vi "MinerHash.vi"(3 "TimeDelay":u32=100, 4 "difficulty":i32=70001, 5 "expected":string="3BE528EC86CE61A4CFCA45749EC9F48BB539D67A", 6 "last_block":string="30644d7a7fdfb0f149224155dad26e06b363a90a") -> (0 "elapsed_time_s":dbl, 1 "duco_numeric_result":i32=70001, 2 "SHA1 string":string="442A0DBBB90711CFDFC0E47CD80FF5F67928C03D")   [LabVIEW 2014]
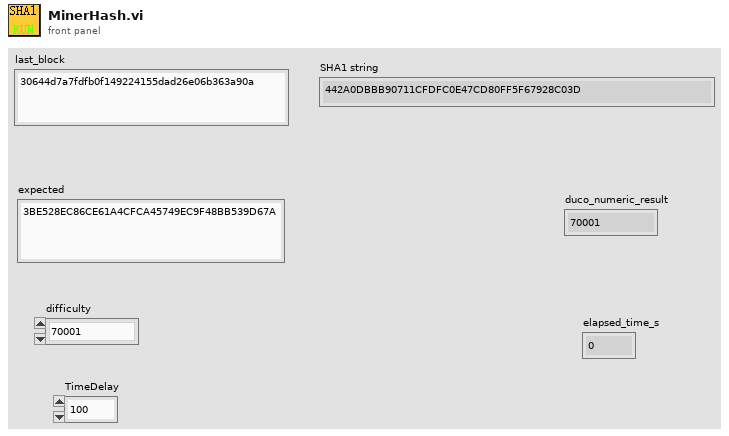
[diagram p1: front panel]
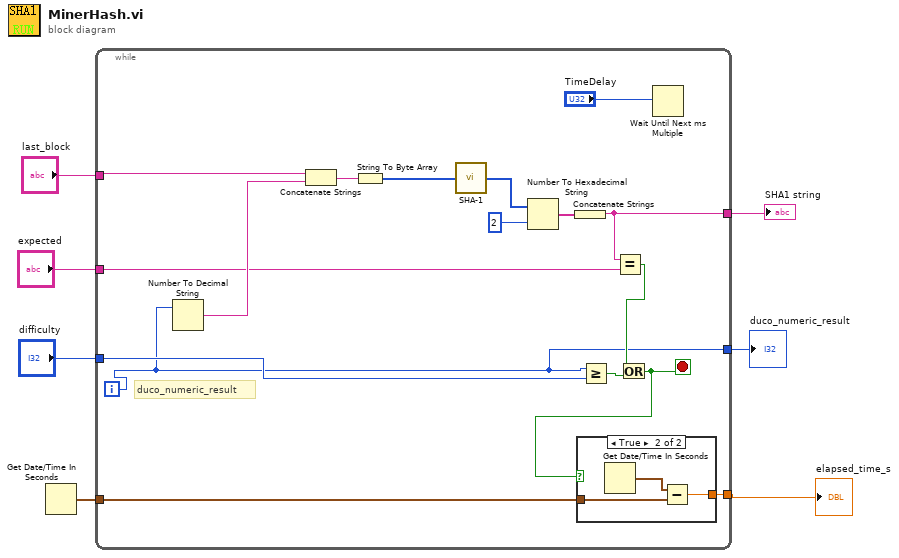
[diagram p0: block diagram]
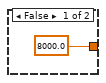
[diagram p2: hidden frame]
diagram:
  n1 = Get Date/Time In Seconds() -> (seconds since 1Jan1904=w2:timestamp)
  n2 = while {
    tunnel: "difficulty" -> [w22]
    tunnel: "last_block" -> [w21]
    tunnel: "expected" -> [w14]
    tunnel: [w12] -> w4
    tunnel: [w11] -> w3
    tunnel: w2 -> [w10]
    tunnel: [w8] -> w1
    i -> [w11]
    stop <- w9 stop-if-true
    # "duco_numeric_result"
    n3 = Number To Decimal String(number=w11) -> (decimal integer string=w16:string)  [unwired: 1 in]
    n4 = Concatenate Strings(w21, w16) -> (w15:string)
    n5 = String To Byte Array(string=w15) -> (unsigned byte array=w17:u8[])
    n6 = call "SHA-1.vi"("Data"=w17) -> ("message-digest"=w18:u8[])
    n7 = Number To Hexadecimal String(1:i16 2 ("width (-)"), 2:w18) -> (0:w20:string[])
    n8 = Concatenate Strings(w20) -> (w12:string)
    n9 = Greater Or Equal?(x=w11, y=w22) -> (x >= y?=w23:bool)
    n10 = Equal?(x=w12, y=w14) -> (x = y?=w13:bool)
    n11 = Or(x=w13, y=w23) -> (x .or. y?=w9:bool)
    n12 = case shown="True" w9 {
      tunnel: w10 -> [_ w28]
      tunnel: [8000.0 w26] -> w8
      frame False {
      }
      frame True {
        n13 = Get Date/Time In Seconds() -> (seconds since 1Jan1904=w27:timestamp)
        n14 = Subtract(x=w27, y=w28) -> (x-y=w26:dbl)
      }
    }
    n15 = Wait Until Next ms Multiple(millisecond multiple="TimeDelay") -> ()  [unwired: 1 out]
  }
  "SHA1 string" <- w4
  "duco_numeric_result" <- w3
  "elapsed_time_s" <- w1
